vi "Set Encoder Type [ENCT].vi"(7 "Micropulse # In":i32, 8 "error in (no error)":errorcluster, 10 "Encoder Type":T1, 11 "Axis No.":u8=1 min=1 max=4) -> (0 "error out":errorcluster, 5 "Micropulse # Out":i32)   [LabVIEW 2026, in "MicroPulse_Driver.lvlib"]
doc: "This command allows the global setting of encoder parameters. Mode 0 is the default mode of 24-bit encoders with the standard output message format. Mode 1 is the full 32-bit output mode. In mode 2 the output mode is full 32 bit but also the output message of inspection modes FLR and FLX/FLZ are now a 32-bit LLC message giving all axis positions instead of the normal LCI message that only gave information about a single axis. Further modes are available 3, 4, and 5 that give the same as modes 0, 1 and 2 but also include with the axis data a message that gives the status of the input/output lines. This message is the same as the reply to an STS 6 command.\n\nThe input mode and filter count are optional parameters. The input mode sets all axis as either full Quadrature or Step/Direction. In Step/Direction the ‘A+’ input is the Step whilst the ‘B+’ is the Direction. Each complete Step pulse is two encoder counts. The filter count is a parameter that can used to clean up the edges of noisy encoders by time hysteresis. This defines the length of time before a decision is made on any input transitions and can filter out noise spikes and noisy level transitions.\nFor individual setting of the Input Mode and Filter Count see the ENCT and ENCF command respectively. It is recommended that these are used.\n\nThe optional fourth parameter (LLC Freq) allows the setting of an increased number of LLC messages (as defined by the Mode parameter above). Normally only one LLC is sent at the start of a data set. If this parameter is used then an LLC will be still sent at the start of a data set, but then further LLC messages will be sent during the data set on before every nth test.\n\nParameters:\n<Mode> : Integer value from 0 to 5:\n0 = 24 Bit output (Default)\n1 = 32 Bit output\n2 = 32 Bit output with LLC message for moving inspection modes\n3 = 24 Bit output with STS 6 message\n4 = 32 Bit output with STS 6 message\n5 = 32 Bit output with LLC message for moving inspection modes with STS 6 message\n\n[Input Mode] : Integer 0 or 1:\n0 = Quadrature (Default)\n1 = Step/Direction\n\n[Filter Count] : Integer value from 0 to 255:\n0 = OFF (Default 0)\n1 to 255 = approximately 100nSec to 20uSec\n\n[LLC Freq] : Integer value \"n\" from 0 to 100 (default 0).\n\nNote:\nThe 32-bit encoders require longer messages for LLC, LCI and LCA. The format is shown in the MicroPulse Output Messages Section.\n\nSystem Compatibility:\nLT1 supports only mode 0 – 2"
uses:
  MicroPulse_Driver.lvlib
  Data/Datatypes/MP - encoder type.ctl
  Private/MP-Registry Action-Enum.ctl
  <instrlib>/Micropulse/Micropulse.lvlib
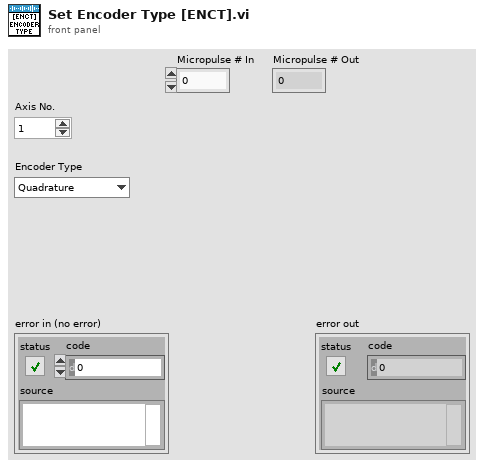
[diagram p1: front panel]
types:
  T1 = typedef "Micropulse.lvlib/MP - encoder type.ctl" = enum16{"Quadrature", "Step/Direction"}
  T2 = typedef "MicroPulse_Driver.lvlib/MP-Registry Action-Enum.ctl" = enum16{"Read", "Add Test", "Add Command", "Add Gate Command", "Add Encoder Command", "Clear Command  List", "Set Registry", "Set System Details", "Set DOF", "Set Velocity", "Disable Asynch Reads", "Enable Asynch Reads", "Add Connection", "Disconnect", "Shutdown"}
  T3 = typedef "Micropulse.lvlib/MP-Registry Data-Cluster.ctl" = cluster{"Instrument Type":T4, "Serial #":u64, "Sample Frequency":T5, "dt (us)":dbl, "DOF":T6, "Material Velocity":dbl, "Asynch Reads":T7, "NUM of Tests":u32, "System Details":T8, "Gates":T10[], "Encoders":T17[], "CMD LUT":variant, "Command List":string}
  T4 = typedef "Micropulse.lvlib/MP - instrument type.ctl" = enum16{"MicroPulse 5", "LT1", "LT2", "LTPA", "MPLT", "MicroPulse 6", "PipeScanner", "<MicroPulse>", "Micropulse 4", "Simulated Data"}
  T5 = typedef "Micropulse.lvlib/MP - sample frequency.ctl" = enum16{"Use Default", "200MHz (LT2 only)", "100MHz", "50MHz", "25MHz", "10MHz"}
  T6 = typedef "Micropulse.lvlib/MP - data output format.ctl" = enum16{"", "8-bit Mode", "10-bit Mode", "12-bit Mode", "16-bit Mode", "8-bit Log Mode", "12-bit Packed Mode"}
  T7 = typedef "Micropulse.lvlib/MP - asynch read mode.ctl" = enum16{"Disabled", "Enabled"}
  T8 = typedef "Micropulse.lvlib/MP - general system status.ctl" = cluster{"System Type":T4, "Serial No.":u64, "Channels":cluster{"Conv":u8, "PA":u16, "Extra":u32}, "Sample Frequency":cluster{"Default":u8, "Actual":u8}, "Software Versions":string, "Data Output Format":cluster{"Default":T6, "Actual":T6}, "Temperatures":cluster{"System":u8, "Processor":u8, "Slave Sys":u8, "Slave Proc":u8}, "Tx Buffer Size":u32, "System Error":string, "No. of Cards":u8, "DAC Gain":i16, "Uptimes":cluster{"since Power":u32, "since RSTS":u32, "since SRST":u32}, "Voltages":cluster{"Nominal":dbl, "Measured":dbl, "Difference":dbl}[], "Interface Cards":T9[]}
  T9 = typedef "Micropulse.lvlib/MP - interface card status.ctl" = cluster{"Status":u8, "Map":u8, "Board - T":u8, "FPGA - T":u8, "PAIF Status":string, "Version":string}
  T10 = typedef "Micropulse.lvlib/MP - Registry Gates.ctl" = cluster{"Display Gate":T11, "ETM Mode":T12, "Echo Gate":T13, "Insp Gates":T14[]}
  T11 = typedef "Micropulse.lvlib/MP - display gate.ctl" = cluster{"Start":dbl, "Length":dbl}
  T12 = typedef "Micropulse.lvlib/MP - echo gate mode.ctl" = enum16{"Echo Trigger OFF", "Echo Gate Display Mode", "Echo Trigger ON", "Multi Gate or FMC Mode", "Reserved", "PA - Echo Trigger ON"}
  T13 = typedef "Micropulse.lvlib/MP - echo gate parameters.ctl" = cluster{"Start (us)":dbl, "Length (us)":dbl, "Threshold":u16, "Colour":u32}
  T14 = typedef "Micropulse.lvlib/MP - multigate inspection gate parameters.ctl" = cluster{"Start (us)":dbl, "Length (us)":dbl, "Threshold":u16, "Enabled?":bool, "Max # Peaks":u16, "Hysteresis":T15, "Mode":T16, "Inverted?":bool, "Colour ":u32}
  T15 = typedef "Micropulse.lvlib/MP - hysteresis level.ctl" = enum16{"None", "3dB", "6dB", "9dB", "12dB"}
  T16 = typedef "Micropulse.lvlib/MP - multigate mode.ctl" = enum16{"1st Peak in Gate", "Largest Peak In Gate", "All Peaks In Gate", "1st Threshold Crossing"}
  T17 = typedef "Micropulse.lvlib/MP - encoder settings.ctl" = cluster{"Encoder Type":T1, "Counts/mm":u32, "Enable Termination?":bool, "Multiplier":u32, "Backlash Period (s)":dbl, "Encoder Filter":u32}
  T18 = typedef "Micropulse.lvlib/TCP config.ctl" = cluster{"Connection ID":refnum<k5>, "IP address":string, "host port":u16, "OC timeout":i32, "Read timeout":i32, "Write timeout":i32}
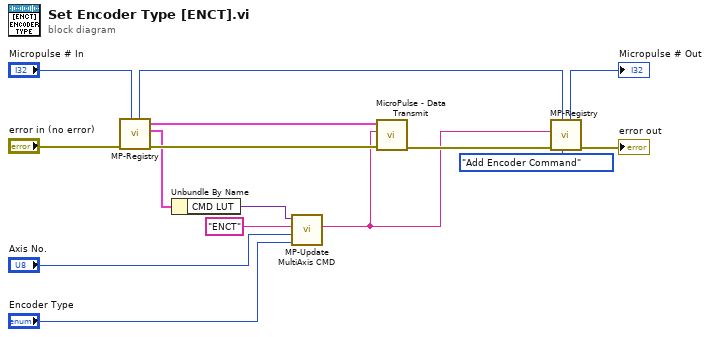
[diagram p0: block diagram]
diagram:
  n1 = call "MP-Registry.vi"("Micropulse # In"="Micropulse # In", "error in (no error)"="error in (no error)") -> ("error out"=w13:errorcluster, "Micropulse Data"=w6:T3, "TCP config"=w12:T18, "Micropulse # Out"=w9:i32)  [unwired: 6 in]
  n2 = Unbundle By Name(w6) -> ("CMD LUT"=w5:variant)
  n3 = call "MP-Update MultiAxis CMD.vi"("Value"="Encoder Type", "Axis No."="Axis No.", "command name"="ENCT" ("name"), "CMD LUT"=w5) -> ("Command out"=w1:string)  [unwired: 7 in]
  n4 = call "MicroPulse - Data Transmit.vi"("error in (no error)"=w13, "data"=w1, "TCP config"=w12) -> ("error out"=w10:errorcluster)  [unwired: 6 in, 2 out]
  n5 = call "MP-Registry.vi"("Action"=MP-Registry_Action-Enum."Add Encoder Command", "Micropulse # In"=w9, "error in (no error)"=w10, "Data in"=w1) -> ("error out"=→"error out":errorcluster, "Micropulse # Out"=→"Micropulse # Out":i32)  [unwired: 4 in, 2 out]
